vi "Get Tunnel Info_MAIN.vi"(7 "Object Placement":enum32{"Choice 1", "Choice 2"}(radio), 8 "error in":errorcluster, 11 "Terminal in":refnum<vi>) -> (0 "error out":errorcluster, 2 "Terminal is on Tunnel":bool, 3 "Terminal Data Cluster":T1)   [LabVIEW 2023]
doc: "Determines if terminal is on a tunnel, and retuns the inner and outer diagram references as well as relative positions for placement of objects with respect to the tunnel position.\n\nWorks on multi-frame and single frame structures as well as flat sequece structures.\n\nThis VI may not provide a valid renum terminal reference, for example is the tunnel is n indexing terminal. If \"Is indexing?\" is true, you must figuer out which of the two terminals is the refnum terminal. There's a VI for that already wrritten called Get Refnum from indexing terminal, which calls this VI for both sides of the terminal and returns the one you want.\n\nIs Refnum? will be false if the terminal contains an array of refnums or clusters. Thus it is only true if it is a useful data type for Bundle Magic to work with.\n\nNote Is tindexing will be true for the tunnel and both of its terminals, and this cannot be used to determine which output is the non-indexing side."
uses:
  <vilib>/Utility/Data Type/NI_Data Type.lvlib
panel:
  out "refnum data type":string
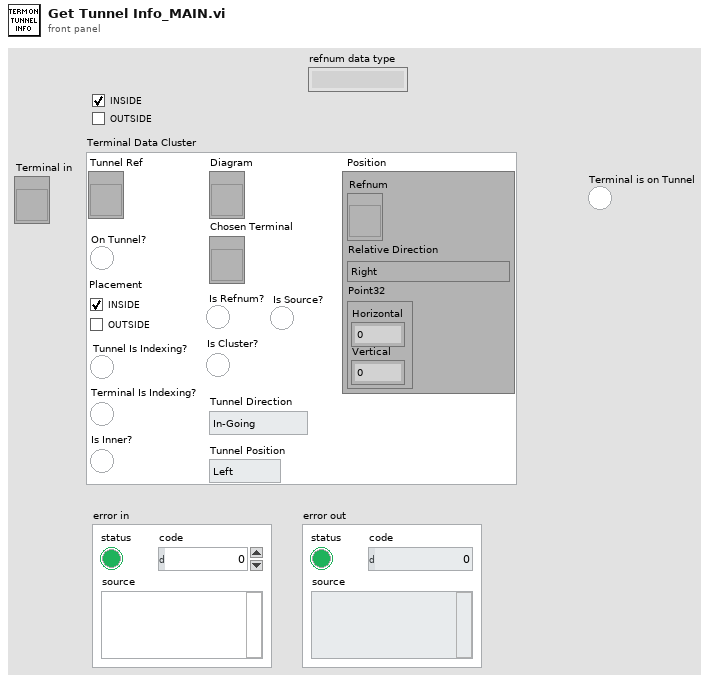
[diagram p1: front panel]
types:
  T1 = cluster{"Tunnel Ref":refnum<vi>, "On Tunnel?":bool, "Placement":enum32{"Choice 1", "Choice 2"}, "Tunnel Is Indexing?":bool, "Diagram":refnum<vi>, "Position":cluster{"Refnum":refnum<vi>, "Relative Direction":enum32{"Right", "Left", "Top", "Bottom", "Top Right", "Top Left", "Bottom Right", "Bottom Left"}, "Point32":cluster{"Horizontal":i32, "Vertical":i32}}, "Chosen Terminal":refnum<vi>, "Is Refnum?":bool, "Is Cluster?":bool, "Is Source?":bool, "Tunnel Direction":enum16{"In-Going", "Out-Going"}, "Tunnel Position":enum16{"Left", "Top", "Right", "Bottom"}, "Is Inner?":bool, "Terminal Is Indexing?":bool}
  T2 = enum8{"Invalid Type", "Void", "I8", "I16", "I32", "I64", "U8", "U16", "U32", "U64", "Single Float", "Double Float", "Extended Float", "Single Complex", "Double Complex", "Extended Complex", "Enum U8", "Enum U16", "Enum U32", "Enum U64", "Single Float With Unit", "Double Float With Unit", "Extended Float With Unit", "Single Complex with Unit", "Double Complex with Unit", "Extended Complex with Unit", "Boolean", "String", "Path", "Picture", "Tag", "Array", "Cluster", "Variant", "LV Variant", "Waveform", "Timestamp", "Digital Waveform", "Digital Data", "ExpressData", "Refnum", "External Data", "VI", "Poly VI", "LabVIEW Class Instance", "Fixed Point"}
  T3 = cluster{"Refnum":refnum<vi>, "Relative Direction":enum32{"Right", "Left", "Top", "Bottom", "Top Right", "Top Left", "Bottom Right", "Bottom Left"}, "Point32":cluster{"Horizontal":i32, "Vertical":i32}}
  T4 = typedef "NI_Data Type.lvlib/Data Type.ctl" = enum8{"Invalid Type", "Void", "I8", "I16", "I32", "I64", "U8", "U16", "U32", "U64", "Single Float", "Double Float", "Extended Float", "Single Complex", "Double Complex", "Extended Complex", "Enum U8", "Enum U16", "Enum U32", "Enum U64", "Single Float With Unit", "Double Float With Unit", "Extended Float With Unit", "Single Complex with Unit", "Double Complex with Unit", "Extended Complex with Unit", "Boolean", "String", "Path", "Picture", "Tag", "Array", "Cluster", "Variant", "LV Variant", "Waveform", "Timestamp", "Digital Waveform", "Digital Data", "ExpressData", "Refnum", "External Data", "VI", "Poly VI", "LabVIEW Class Instance", "Fixed Point", "Set Collection", "Map Collection"}
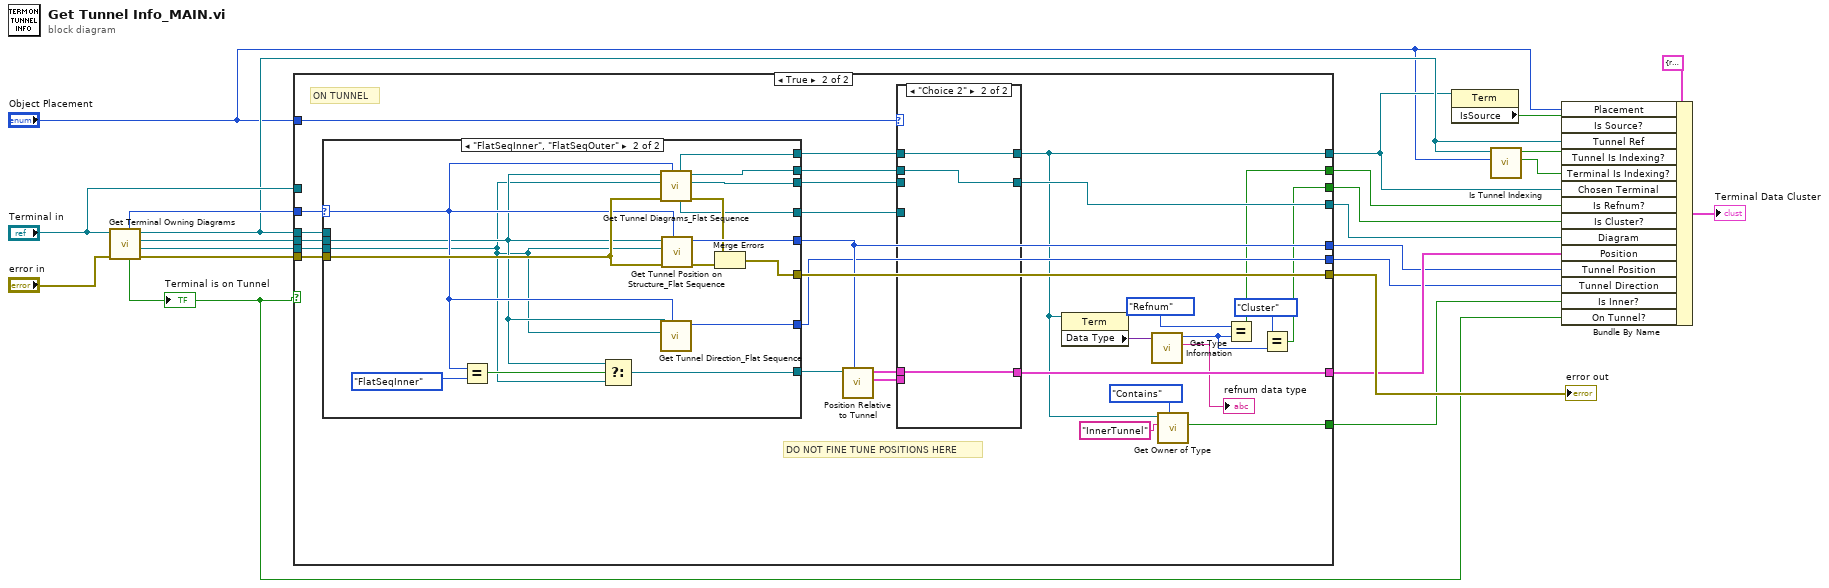
[diagram p0: block diagram]
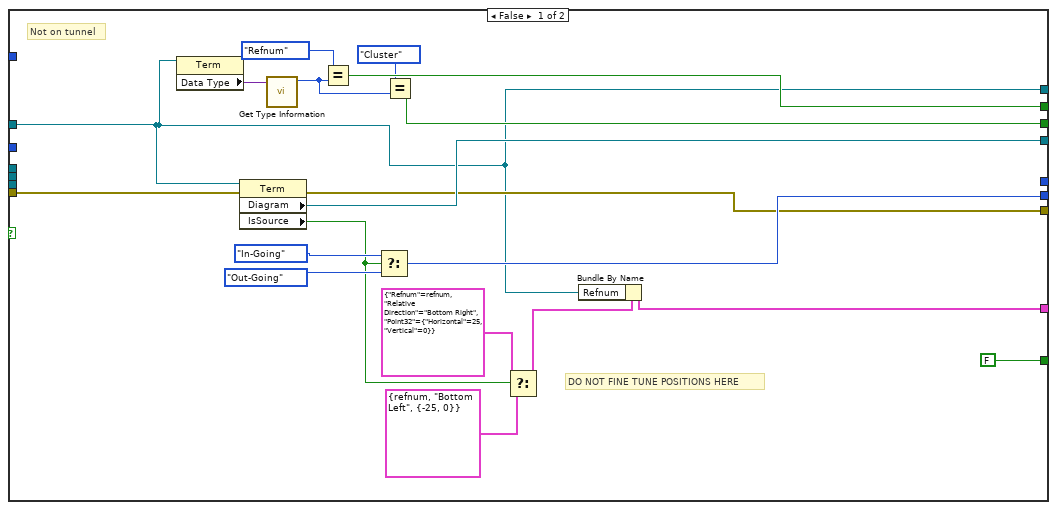
[diagram p2: hidden frame]
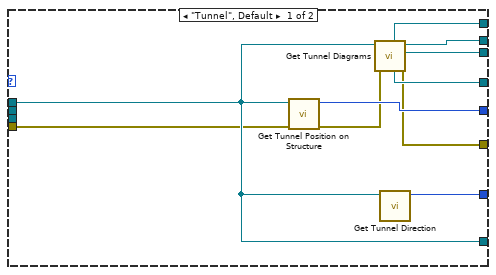
[diagram p4: hidden frame]
diagram:
  n1 = call "Get Terminal Owning Diagrams.vi"("error in (no error)"="error in", "Terminal in"="Terminal in") -> ("error out"=w19:errorcluster, "FlatSeqOutTun Refnum"=w22:refnum<vi>, "FlatSeqInTun Refnum"=w21:refnum<vi>, "Tunnel Ref"=w6:refnum<vi>, "Terminal is on Tunnel"=w1:bool, "Tunnel Type"=w20:enum16{"Tunnel", "FlatSeqInner", "FlatSeqOuter"})  [unwired: 3 in, 1 out]
  "Terminal is on Tunnel" <- w1
  n2 = case shown="True" w1 {
    tunnel: [w36 w71] -> w23
    tunnel: w22 -> [_ w70]
    tunnel: w21 -> [_ w69]
    tunnel: w20 -> [_ w68]
    tunnel: w19 -> [w35 w67]
    tunnel: [w42 w55] -> w17
    tunnel: [w25 w45] -> w5
    tunnel: [_ w66] -> w12
    tunnel: [w40 w65] -> w11
    tunnel: w6 -> [_ w64]
    tunnel: "Terminal in" -> [w25 _]
    tunnel: [w32 w58] -> w13
    tunnel: "Object Placement" -> [_ w63]
    tunnel: [w29 w51] -> w9
    tunnel: [w26 w48] -> w8
    tunnel: [FALSE w44] -> w7
    frame False {
      # "Not on tunnel"
      # "DO NOT FINE TUNE POSITIONS HERE"
      n3 = property class="Term"(reference=w25) -> ("Data Type"=w31:variant)  [unwired: 1 in, 2 out]
      n4 = property class="Term"(reference=w25, error in=w35) -> (error out=w36:errorcluster, "Diagram"=w42:refnum<vi>, "IsSource"=w34:bool)  [unwired: 1 out]
      n5 = call <vilib>:"Get Type Information.vi"("variant"=w31) -> ("type"=w27:T4)  [unwired: 6 in, 4 out]
      n6 = Equal?(x=T2."Refnum" ("type"), y=w27) -> (x = y?=w29:bool)
      n7 = Select(t=enum16{"In-Going", "Out-Going"}."In-Going" ("Tunnel Direction"), s=w34, f=enum16{"In-Going", "Out-Going"}."Out-Going" ("Tunnel Direction")) -> (s? t:f=w40:enum16{"In-Going", "Out-Going"})
      n8 = Equal?(x=T2."Cluster" ("type"), y=w27) -> (x = y?=w26:bool)
      n9 = Select(t=T3 {"Refnum"=refnum, "Relative Direction"=enum."Bottom Right", "Point32"={"Horizontal"=25, "Vertical"=0}} ("Outer Position"), s=w34, f=T3 {"Refnum"=refnum, "Relative Direction"=enum."Bottom Left", "Point32"={"Horizontal"=-25, "Vertical"=0}} ("Outer Position")) -> (s? t:f=w33:T3)
      n10 = Bundle By Name(cluster=w33, "Refnum"=w25) -> (w32:T3)
    }
    frame True {
      # "DO NOT FINE TUNE POSITIONS HERE"
      # "ON TUNNEL"
      n11 = case shown="\"FlatSeqInner\", \"FlatSeqOuter\"" w68 {
        selector: w68 -> [_ w95]
        tunnel: w67 -> [w80 w100]
        tunnel: [w78 w97] -> w71
        tunnel: [w87 w103] -> w61
        tunnel: [w86 w102] -> w59
        tunnel: w64 -> [w83 _]
        tunnel: [w85 w96] -> w65
        tunnel: [w84 w101] -> w66
        tunnel: w69 -> [_ w92]
        tunnel: w70 -> [_ w91]
        tunnel: [w83 w90] -> w54
        tunnel: [w82 w89] -> w62
        tunnel: [w81 w88] -> w60
        frame "Tunnel", Default {
          n12 = call "Get Tunnel Position on Structure.vi"("error in"=w80, "Tunnel Ref"=w83) -> ("error out"=w79:errorcluster, "Tunnel Position"=w84:enum16{"Left", "Top", "Right", "Bottom"})  [unwired: 6 in, 2 out]
          n13 = call "Get Tunnel Diagrams.vi"("error in"=w79, "Tunnel in"=w83) -> ("error out"=w78:errorcluster, "Inner Diagram"=w86:refnum<vi>, "Outer Diagram"=w87:refnum<vi>, "Inner Terminal"=w81:refnum<vi>, "Outer Terminal"=w82:refnum<vi>)  [unwired: 4 in, 1 out]
          n14 = call "Get Tunnel Direction.vi"("Tunnel in"=w83) -> ("Tunnel Direction"=w85:enum16{"In-Going", "Out-Going"})  [unwired: 10 in]
        }
        frame "FlatSeqInner", "FlatSeqOuter" {
          n15 = Equal?(x=w95, y=enum16{"Tunnel", "FlatSeqInner", "FlatSeqOuter"}."FlatSeqInner" ("Tunnel Type")) -> (x = y?=w93:bool)
          n16 = Select(t=w92, s=w93, f=w91) -> (s? t:f=w90:refnum<vi>)
          n17 = call "Get Tunnel Diagrams_Flat Sequence.vi"("Tunnel Type"=w95, "error in"=w100, "FlatSeqOutTun Refnum"=w91, "FlatSeqInTun Refnum"=w92) -> ("error out"=w99:errorcluster, "Inner/Right Diagram"=w102:refnum<vi>, "Outer/Left Diagram"=w103:refnum<vi>, "Inner/Right Terminal"=w88:refnum<vi>, "Outer/Left Terminal"=w89:refnum<vi>)  [unwired: 2 in, 1 out]
          n18 = call "Get Tunnel Direction_Flat Sequence.vi"("Tunnel Type"=w95, "FlatSeqOutTun Refnum"=w91, "FlatSeqInTun Refnum"=w92) -> ("Tunnel Direction"=w96:enum16{"In-Going", "Out-Going"})  [unwired: 8 in]
          n19 = call "Get Tunnel Position on Structure_Flat Sequence.vi"("Tunnel Type"=w95, "error in"=w100, "FlatSeqOutTun Refnum"=w91, "FlatSeqInTun Refnum"=w92) -> ("error out"=w98:errorcluster, "Tunnel Position"=w101:enum16{"Left", "Top", "Right", "Bottom"})  [unwired: 5 in, 1 out]
          n20 = Merge Errors(w99, w98) -> (w97:errorcluster)
        }
      }
      n21 = call "Position Relative to Tunnel.vi"("Tunnel Position"=w66, "Tunnel in"=w54) -> ("Inner Position"=w57:T3, "Outer Position"=w56:T3)  [unwired: 8 in]
      n22 = case shown="\"Choice 2\"" w63 {
        tunnel: [w74 w77] -> w45
        tunnel: w62 -> [_ w77]
        tunnel: [w73 w76] -> w55
        tunnel: w61 -> [_ w76]
        tunnel: w60 -> [w74 _]
        tunnel: w59 -> [w73 _]
        tunnel: [w72 w75] -> w58
        tunnel: w57 -> [w72 _]
        tunnel: w56 -> [_ w75]
        frame "Choice 1", Default {
        }
        frame "Choice 2" {
        }
      }
      n23 = property class="Term"(reference=w45) -> ("Data Type"=w53:variant)  [unwired: 1 in, 2 out]
      n24 = call <vilib>:"Get Type Information.vi"("variant"=w53) -> ("name"=→"refnum data type":string, "type"=w50:T4)  [unwired: 6 in, 3 out]
      n25 = call "Get Owner of Type.vi"("Match Type"=enum16{"Exact Match", "Contains"}."Contains", "Owner Class Name desired"="InnerTunnel", "reference"=w45) -> ("Owner of type found?"=w44:bool)  [unwired: 4 in, 4 out]
      n26 = Equal?(x=T2."Refnum" ("type"), y=w50) -> (x = y?=w51:bool)
      n27 = Equal?(x=T2."Cluster" ("type"), y=w50) -> (x = y?=w48:bool)
    }
  }
  "error out" <- w23
  n28 = property class="Term"(reference=w5) -> ("IsSource"=w10:bool)  [unwired: 1 in, 2 out]
  n29 = call "Is Tunnel Indexing.vi"("Object Placement"="Object Placement", "Tunnel Ref"=w6) -> ("Chosen Terminal is indexing"=w2:bool, "Tunnel is indexing"=w3:bool)  [unwired: 4 in, 4 out]
  n30 = Bundle By Name(cluster=T1 {"Tunnel Ref"=refnum, "On Tunnel?"=FALSE, "Placement"=enum."Choice 1", "Tunnel Is Indexing?"=FALSE, "Diagram"=refnum, "Position"={"Refnum"=refnum, "Relative Direction"=enum."Right", "Point32"={"Horizontal"=0, "Vertical"=0}}, "Chosen Terminal"=refnum, "Is Refnum?"=FALSE, "Is Cluster?"=FALSE, "Is Source?"=FALSE, "Tunnel Direction"=enum."In-Going", "Tunnel Position"=enum."Left", "Is Inner?"=FALSE, "Terminal Is Indexing?"=FALSE} ("Tunnel Data Cluster"), "Placement"="Object Placement", "Is Source?"=w10, "Tunnel Ref"=w6, "Tunnel Is Indexing?"=w3, "Terminal Is Indexing?"=w2, "Chosen Terminal"=w5, "Is Refnum?"=w9, "Is Cluster?"=w8, "Diagram"=w17, "Position"=w13, "Tunnel Position"=w12, "Tunnel Direction"=w11, "Is Inner?"=w7, "On Tunnel?"=w1) -> (→"Terminal Data Cluster":T1)
